vi "Condition Msg Msg VI.vi"(6 "Name":string, 8 "error in":errorcluster, 9 "Conn Pane Terminals.Msg Output Indicator":i32[](array[numeric]), 10 "Name Msg Refs.Msg VI":refnum<vi>) -> (0 "error out":errorcluster)   [LabVIEW 2025, in "_Msg Rescript.lvlib" / "_Msg Rescript.lvclass"]
uses:
  _Msg Rescript.lvclass
  _Msg Rescript.lvclass/_Msg Rescript.ctl
  <vilib>/Utility/traverseref.llb/TRef TravTarget.ctl
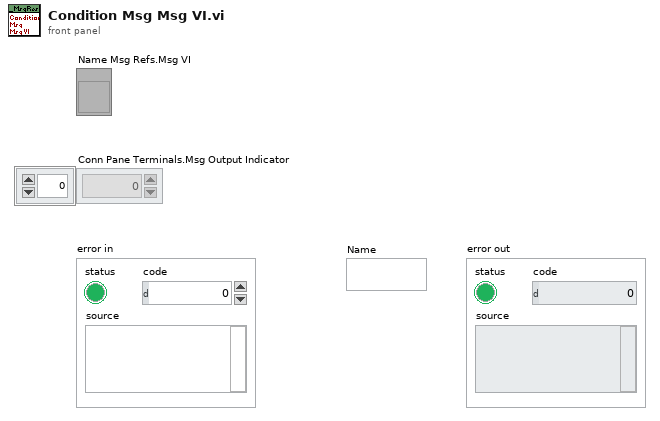
[diagram p1: front panel]
types:
  T1 = typedef "TRef TravTarget.ctl" = enum16{"FP", "BD", "Other"}
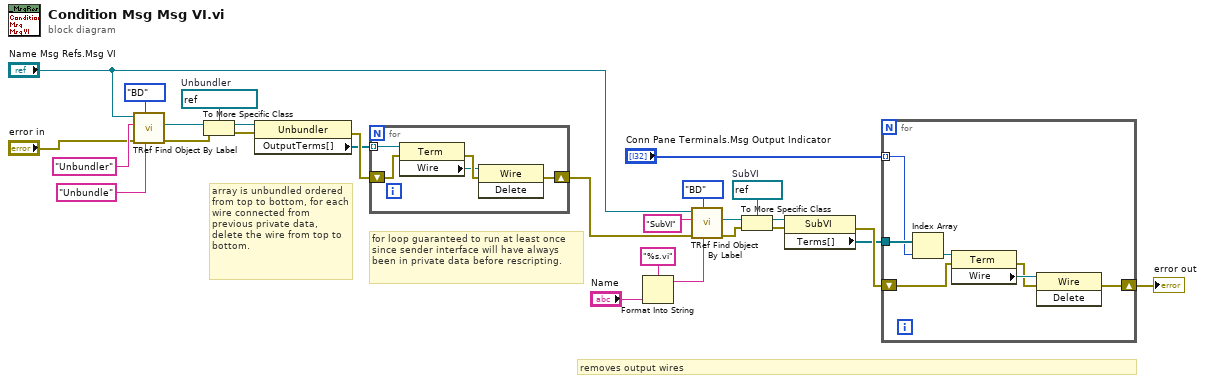
[diagram p0: block diagram]
diagram:
  w15 = refnum<vi> refnum  # SubVI
  w25 = refnum<vi> refnum  # Unbundler
  # "removes output wires"
  # "for loop guaranteed to run at least once since sender interface will have always been in private data before rescripting."
  # "array is unbundled ordered from top to bottom, for each wire connected from previous private data, delete the wire from top to bottom."
  n1 = call <vilib>:"TRef Find Object By Label.vi"("Label"="Unbundle", "Traverse Target"=TRef_TravTarget."BD", "error in (no error)"="error in", "Class Name"="Unbundler", "VI Ref"="Name Msg Refs.Msg VI") -> ("error out"=w26:errorcluster, "Found Obj Ref"=w24:refnum<vi>)  [unwired: 3 in, 2 out]
  n2 = To More Specific Class(target class=w25, reference=w24, error in=w26) -> (specific class reference=w21:refnum<vi>, error out=w19:errorcluster)
  n3 = property class="Unbundler"(reference=w21, error in=w19) -> (error out=w27:errorcluster, "OutputTerms[]"=w17:refnum<vi>[])  [unwired: 1 out]
  n4 = for {
    shift-right: [w28] -> w3
    shift-left: w27 -> [w29]
    tunnel: w17 -> [w31] mode=indexing
    n5 = property class="Term"(reference=w31, error in=w29) -> (error out=w32:errorcluster, "Wire"=w30:refnum<vi>)  [unwired: 1 out]
    n6 = invoke class="Wire" method="Delete"(reference=w30, error in=w32) -> (error out=w28:errorcluster)  [unwired: 1 in, 2 out]
  }
  n7 = Format Into String(format string="%s.vi", "Name") -> (resulting string=w6:string)  [unwired: 2 in, 1 out]
  n8 = call <vilib>:"TRef Find Object By Label.vi"("Label"=w6, "Traverse Target"=TRef_TravTarget."BD", "error in (no error)"=w3, "Class Name"="SubVI", "VI Ref"="Name Msg Refs.Msg VI") -> ("error out"=w14:errorcluster, "Found Obj Ref"=w8:refnum<vi>)  [unwired: 3 in, 2 out]
  n9 = To More Specific Class(target class=w15, reference=w8, error in=w14) -> (specific class reference=w12:refnum<vi>, error out=w11:errorcluster)
  n10 = property class="SubVI"(reference=w12, error in=w11) -> (error out=w10:errorcluster, "Terms[]"=w5:refnum<vi>[])  [unwired: 1 out]
  n11 = for {
    tunnel: w5 -> [w39]
    tunnel: "Conn Pane Terminals.Msg Output Indicator" -> [w38] mode=indexing
    shift-right: [w37] -> w1
    shift-left: w10 -> [w34]
    n12 = Index Array(array=w39, index=w38) -> (element=w36:refnum<vi>)
    n13 = property class="Term"(reference=w36, error in=w34) -> (error out=w33:errorcluster, "Wire"=w35:refnum<vi>)  [unwired: 1 out]
    n14 = invoke class="Wire" method="Delete"(reference=w35, error in=w33) -> (error out=w37:errorcluster)  [unwired: 1 in, 2 out]
  }
  "error out" <- w1
